vi "Read POV Polymorphic.vi"   [LabVIEW 2010, in "FTC.lvlib" / "Remote Interface.lvlib"]
uses:
  Remote Interface.lvlib
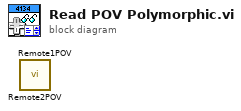
[diagram p0: block diagram]
diagram:
  n1 = call "Remote2POV.vi"() -> ()  [unwired: 5 in, 1 out]
  n2 = call "Remote1POV.vi"() -> ()  [unwired: 5 in, 1 out]
